vi "readProtocol.vi"(8 "error in (no error)":errorcluster, 11 "TCP Network Connection in":refnum<k5>) -> (0 "error out":errorcluster, 1 "data out":string)   [LabVIEW 2019, in "ESP301viaTCPIP.lvlib"]
uses:
  ESP301viaTCPIP.lvlib
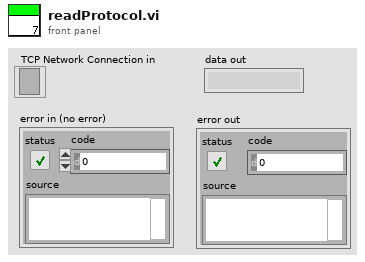
[diagram p1: front panel]
types:
  T1 = enum16{"Standard", "Buffered", "CRLF", "Immediate"}
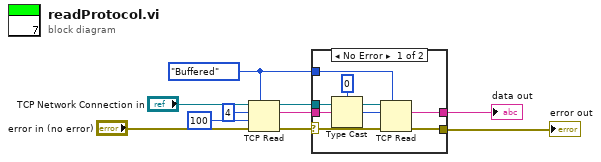
[diagram p0: block diagram]
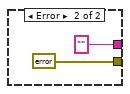
[diagram p2: hidden frame]
diagram:
  w10 = T1."Buffered" ("mode (standard)")
  n1 = TCP Read(connection ID="TCP Network Connection in", bytes to read=4, error in (no error)="error in (no error)", 7:w10, 9:100 ("timeout ms (25000)")) -> (connection ID out=w5:refnum<k5>, data out=w6:string, error out=w1:errorcluster)
  n2 = case shown="No Error" w1 {
    selector: w1 -> [w11 _]
    tunnel: w10 -> [w18 _]
    tunnel: w6 -> [w15 _]
    tunnel: w5 -> [w14 _]
    tunnel: [w13 errorcluster {"status"=FALSE, "code"=0, "source"=""} ("error out")] -> w3
    tunnel: [w12 "" ("data out")] -> w2
    frame No Error {
      n3 = Type Cast(type=0, x=w15) -> (*(type *) &x=w17:i32)
      n4 = TCP Read(connection ID=w14, bytes to read=w17, error in (no error)=w11, 7:w18) -> (data out=w12:string, error out=w13:errorcluster)  [unwired: 1 in, 1 out]
    }
    frame Error {
    }
  }
  "data out" <- w2
  "error out" <- w3
